vi "FindUniqueNodeName.vi"(10 "Node Name":string, 11 "Parent Node In":refnum<data-value>) -> (2 "Unique Node Name Out":string, 3 "Parent Node Out":refnum<data-value>)   [LabVIEW 2019]
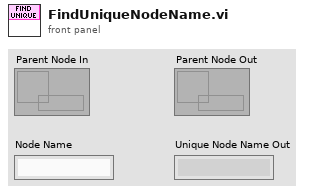
[diagram p1: front panel]
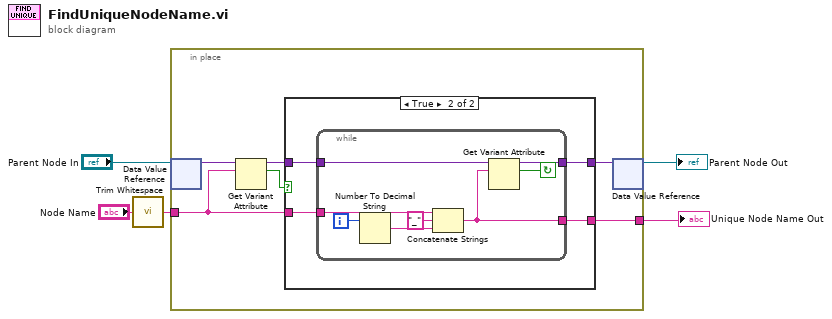
[diagram p0: block diagram]
diagram:
  n1 = call <vilib>:"Trim Whitespace.vi"("string"="Node Name") -> ("trimmed string"=w1:string)  [unwired: 1 in]
  n2 = in-place {
    in-place-border: w1 -> [w7]
    in-place-border: [w11] -> w5
    n3 = in-place-dvr #1("Parent Node In") -> (w9:variant)  [unwired: 1 out]
    n4 = Get Variant Attribute(Variant=w9, name=w7) -> (duplicate Variant=w8:variant, found=w6:bool)  [unwired: 2 in, 2 out]
    n5 = case shown="True" w6 {
      tunnel: [w12 w17] -> w11
      tunnel: [w13 w16] -> w10
      tunnel: w8 -> [w13 w15]
      tunnel: w7 -> [w12 w14]
      frame False {
      }
      frame True {
        n6 = while {
          tunnel: w15 -> [w21]
          tunnel: w14 -> [w23]
          tunnel: [w19] -> w17
          tunnel: [w18] -> w16
          i -> [w25]
          stop <- w20 continue-if-true
          n7 = Number To Decimal String(number=w25) -> (decimal integer string=w22:string)  [unwired: 1 in]
          n8 = Concatenate Strings(w23, "_" ("string"), w22) -> (w19:string)
          n9 = Get Variant Attribute(Variant=w21, name=w19) -> (duplicate Variant=w18:variant, found=w20:bool)  [unwired: 2 in, 2 out]
        }
      }
    }
    n10 = in-place-dvr #1(w10) -> (→"Parent Node Out":refnum<data-value>)  [unwired: 1 out]
  }
  "Unique Node Name Out" <- w5
